vi "PCO_SetRecordingStruct.vi"(8 "error in (no error)":errorcluster, 11 "Handle":u64) -> (0 "error out":errorcluster, 3 "Handle Out":u64, 5 "return type":u32 format="%x")   [LabVIEW 2011]
uses:
  SC2_Cam64.dll
panel:
  in  "PCO_Recording":T1
  out "PCO_Recording":u16[](array[numeric])
  # "does not work!!"
  # "A00A3001"
  # "NOT tested"
  # "! dw Order is different!?"
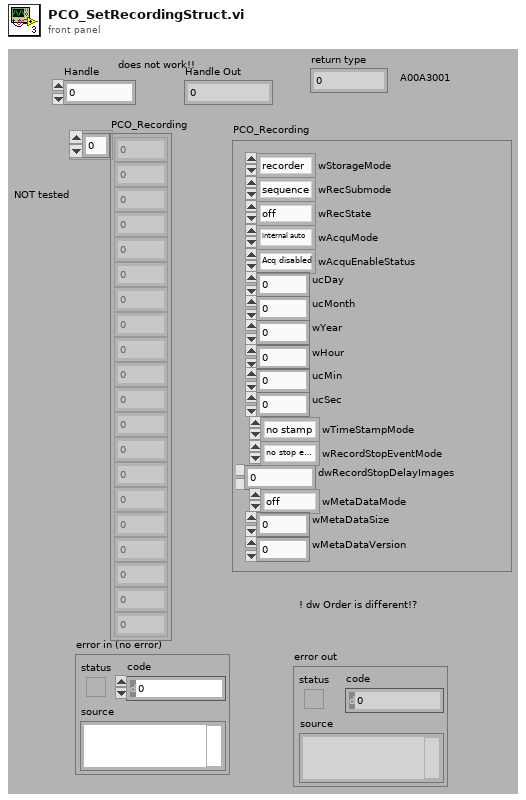
[diagram p1: front panel]
types:
  T1 = cluster{"wStorageMode":enum16{"recorder", "fifo"}, "wRecSubmode":enum16{"sequence", "ringbuffer"}, "wRecState":enum16{"off", "on"}, "wAcquMode":enum16{"internal auto", "external"}, "wAcquEnableStatus":enum16{"Acq disabled", "enalbled"}, "ucDay":u8, "ucMonth":u8, "wYear":u16, "wHour":u16, "ucMin":u8, "ucSec":u8, "wTimeStampMode":enum16{"no stamp", "stamp in first 14 pixel", "stamp+ASCII"}, "wRecordStopEventMode":enum16{"no stop event recording", "recording stops with event"}, "dwRecordStopDelayImages":u32, "wMetaDataMode":enum16{"off", "on"}, "wMetaDataSize":u16, "wMetaDataVersion":u16}
  T2 = cluster{"wStorageMode":u16, "wRecSubmode":u16, "wRecState":u16, "wAcquMode":u16, "wAcquEnableStatus":u16, "ucDay":u8, "ucMonth":u8, "wYear":u16, "wHour":u16, "ucMin":u8, "ucSec":u8, "wTimeStampMode":u16, "wRecordStopEventMode":u16, "dwRecordStopDelayImages":u32, "wMetaDataMode":u16, "wMetaDataSize":u16, "wMetaDataVersion":u16}
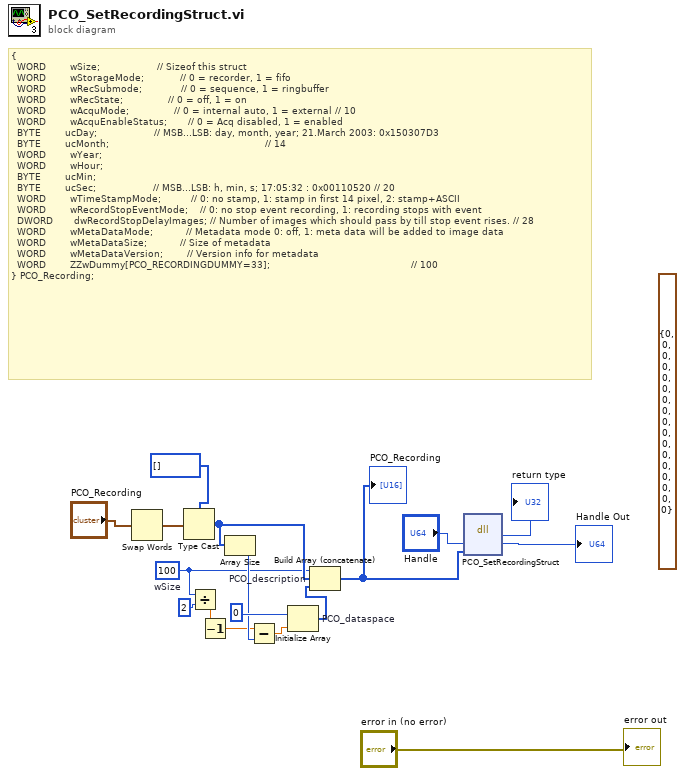
[diagram p0: block diagram]
diagram:
  (unwired) T2 {"wStorageMode"=0, "wRecSubmode"=0, "wRecState"=0, "wAcquMode"=0, "wAcquEnableStatus"=0, "ucDay"=0, "ucMonth"=0, "wYear"=0, "wHour"=0, "ucMin"=0, "ucSec"=0, "wTimeStampMode"=0, "wRecordStopEventMode"=0, "dwRecordStopDelayImages"=0, "wMetaDataMode"=0, "wMetaDataSize"=0, "wMetaDataVersion"=0} ("PCO_Recording")
  w4 = u16 100  # wSize
  # "{\n  WORD        wSize;                   // Sizeof this struct\n  WORD        wStorageMode;            // 0 = recorder, 1 = fifo\n  WORD        wRecSubmode;             // 0 = sequence, 1 = ringbuffer\n  WORD        wRecState;               // 0 = off, 1 = on\n  WORD        wAcquMode;               // 0 = internal auto, 1 = external // 10\n  WORD        wAcquEnableStatus;       // 0 = Acq disabled, 1 = enabled\n  BYTE        ucDay;                   // MSB...LSB: day, month, year; 21.March 2003: 0x150307D3\n  BYTE        ucMonth;                                                    // 14\n  WORD        wYear;\n  WORD        wHour;\n  BYTE        ucMin;\n  BYTE        ucSec;                   // MSB...LSB: h, min, s; 17:05:32 : 0x00110520 // 20\n  WORD        wTimeStampMode;          // 0: no stamp, 1: stamp in first 14 pixel, 2: stamp+ASCII\n  WORD        wRecordStopEventMode;    // 0: no stop event recording, 1: recording stops with event\n  DWORD       dwRecordStopDelayImages; // Number of images which should pass by till stop event rises. // 28\n  WORD        wMetaDataMode;           // Metadata mode 0: off, 1: meta data will be added to image data\n  WORD        wMetaDataSize;           // Size of metadata\n  WORD        wMetaDataVersion;        // Version info for metadata\n  WORD        ZZwDummy[PCO_RECORDINGDUMMY=33];                                               // 100\n} PCO_Recording;"
  n1 = Swap Words(1:"PCO_Recording") -> (0:w9:T2)
  n2 = Type Cast(type=u16[] [], x=w9) -> (*(type *) &x=w7:u16[])
  n3 = Divide(x=w4, y=u16 2) -> (x/y=w11:dbl)
  n4 = Decrement(x=w11) -> (x-1=w3:dbl)
  n5 = Array Size(array=w7) -> (size(s)=w6:i32)
  n6 = Subtract(x=w3, y=w6) -> (x-y=w2:dbl)
  n7 = Initialize Array "PCO_dataspace"(u16 0 ("element"), w2) -> (w5:u16[])
  n8 = Build Array (concatenate) "PCO_description"(w4, w7, w5) -> (w1:u16[])
  "PCO_Recording" <- w1
  n9 = dll-call lib="SC2_Cam*.*" fn="PCO_SetRecordingStruct"("Handle"="Handle", "PCO_Recording"=w1) -> ("return type"=→"return type":u32, "Handle"=→"Handle Out":u64)  [unwired: 4 in, 2 out]
  "error out" <- "error in (no error)"
